vi "AlliGator Pseudo Dirac IRF.vi"(8 "Error In":errorcluster, 9 "Decay Bin Size":dbl[unit], 10 "Period":dbl[unit], 11 "Reference Decay in":cluster{"t Array":dbl[], "IRF Array":dbl[]}) -> (0 "Error Out":errorcluster, 3 "Reference Decay out":cluster{"t Array":dbl[], "IRF Array":dbl[]})   [LabVIEW 2021, in "AlliGator Fit Method Benchmark.lvlib"]
doc: "Computes a decay with a single non-zero bin."
uses:
  AlliGator Fit Method Benchmark.lvlib
  Arrays/Linear Ramp End Options.ctl
  43802517-97f2-45ec-b194-7fc90ec129af.vi
  631369a9-f018-4919-9878-7582767838ef.vi
  <vilib>/Utility/error.llb/Error Cluster From Error Code.vi
  <vilib>/ErrorRing/Error Ring.xnode
  Arrays/Arrays.lvlib
panel:
  # "see the AlliGator License on the block diagram (Ctrl+E or Window:Show Block Diagram)"
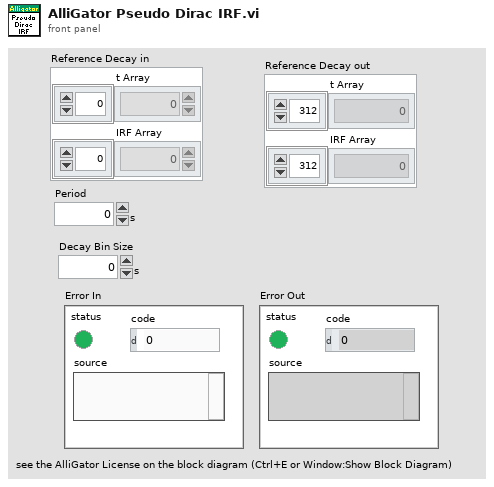
[diagram p1: front panel]
types:
  T1 = typedef "Arrays.lvlib/Linear Ramp End Options.ctl" = enum16{"Include Min/Exclude Max", "Exclude Min/Include Max", "Include Both Ends", "Exclude Both Ends"}
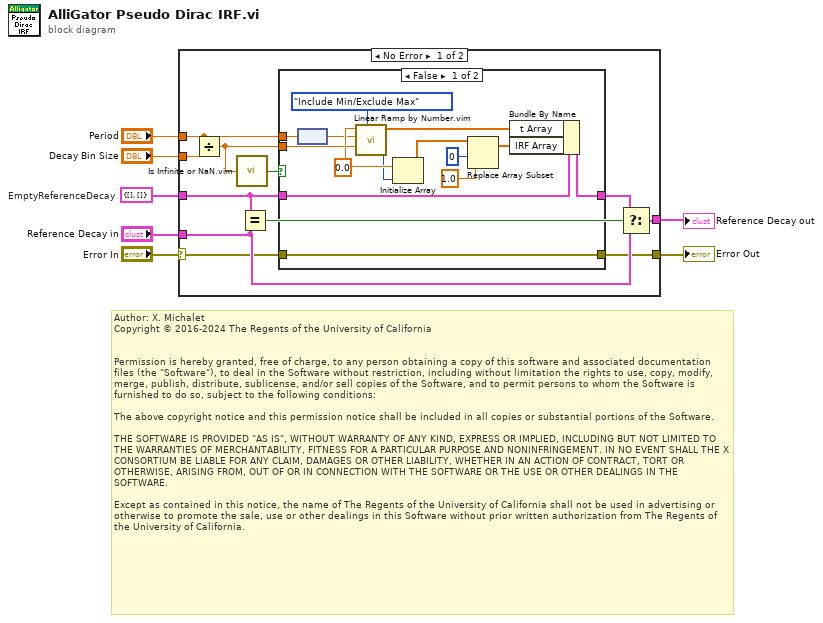
[diagram p0: block diagram]
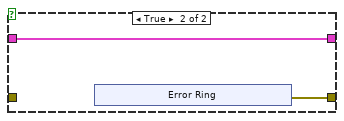
[diagram p2: hidden frame]
diagram:
  w3 = cluster{"t Array":dbl[], "IRF Array":dbl[]} {"t Array"=[], "IRF Array"=[]}  # EmptyReferenceDecay
  # "Author: X. Michalet\nCopyright © 2016-2024 The Regents of the University of California\n \n\nPermission is hereby granted, free of charge, to any person obtaining a copy of this software and associated documentation files (the \"Software\"), to deal in the Software without restriction, including without limitation the rights to use, copy, modify, merge, publish, distribute, sublicense, and/or sell copies of the Software, and to permit persons to whom the Software is furnished to do so, subject to the following conditions:\n\nThe above copyright notice and this permission notice shall be included in all copies or substantial portions of the Software.\n\nTHE SOFTWARE IS PROVIDED \"AS IS\", WITHOUT WARRANTY OF ANY KIND, EXPRESS OR IMPLIED, INCLUDING BUT NOT LIMITED TO THE WARRANTIES OF MERCHANTABILITY, FITNESS FOR A PARTICULAR PURPOSE AND NONINFRINGEMENT. IN NO EVENT SHALL THE X CONSORTIUM BE LIABLE FOR ANY CLAIM, DAMAGES OR OTHER LIABILITY, WHETHER IN AN ACTION OF CONTRACT, TORT OR OTHERWISE, ARISING FROM, OUT OF OR IN CONNECTION WITH THE SOFTWARE OR THE USE OR OTHER DEALINGS IN THE SOFTWARE.\n\nExcept as contained in this notice, the name of The Regents of the University of California shall not be used in advertising or otherwise to promote the sale, use or other dealings in this Software without prior written authorization from The Regents of the University of California."
  n1 = case shown="No Error" "Error In" {
    selector: "Error In" -> [w8 w40]
    tunnel: "Reference Decay in" -> [w17 w39]
    tunnel: [w16 w39] -> w6
    tunnel: "Decay Bin Size" -> [w15 _]
    tunnel: "Period" -> [w12 _]
    tunnel: w3 -> [w11 _]
    tunnel: [w9 w40] -> w1
    frame No Error {
      n2 = Divide(x=w12, y=w15) -> (x/y=w14:dbl)
      n3 = call "Is Infinite or NaN.vim"("Number"=w14) -> ("Is NaN or Inf?"=w13:bool)  [unwired: 8 in]
      n4 = Equal?(x=w11, y=w17) -> (x = y?=w18:bool)
      n5 = case shown="False" w13 {
        tunnel: w14 -> [w29 _]
        tunnel: w12 -> [w27 _]
        tunnel: w11 -> [w24 w34]
        tunnel: [w21 w34] -> w10
        tunnel: [w20 w33] -> w9
        tunnel: w8 -> [w20 _]
        frame False {
          w28 = 0.0 ("element")
          n6 = node(w27) -> (w26:dbl)
          n7 = call "Linear Ramp by Number.vim"("Options"=Linear_Ramp_End_Options."Include Min/Exclude Max", "# Steps (1)"=w29, "End (1)"=w26, "Start (0)"=w28) -> ("# Elements"=w19:i32, "Ramp"=w23:dbl[])  [unwired: 5 in, 1 out]
          n8 = Initialize Array(w28, w19) -> (w32:dbl[])
          n9 = Replace Array Subset(array=w32, new element=1.0 ("new element/subarray"), index=0) -> (w22:dbl[])
          n10 = Bundle By Name(cluster=w24, "t Array"=w23, "IRF Array"=w22) -> (w21:cluster{"t Array":dbl[], "IRF Array":dbl[]})
        }
        frame True {
          n11 = xnode "Error Ring"() -> ("error out"=w33:errorcluster)
        }
      }
      n12 = Select(t=w10, s=w18, f=w17) -> (s? t:f=w16:cluster{"t Array":dbl[], "IRF Array":dbl[]})
    }
    frame Error {
    }
  }
  "Reference Decay out" <- w6
  "Error Out" <- w1
